vi "Disconnect.vi"(8 "error in":errorcluster, 11 "Luminos in":refnum<class "Luminos.lvclass">) -> (0 "error out":errorcluster, 3 "Luminos out":refnum<class "Luminos.lvclass">)   [LabVIEW 2018, in "Luminos.lvlib" / "Luminos.lvclass"]
uses:
  Luminos.lvclass
  PPLs/Axis/Axis.lvlibp/Axis.lvclass
  <instrlib>/ZaberTSeries/ZaberTSeries.lvlib
  C:/Projects/LabVIEW/PPLs/Axis/Axis.lvlibp/Axis.lvclass
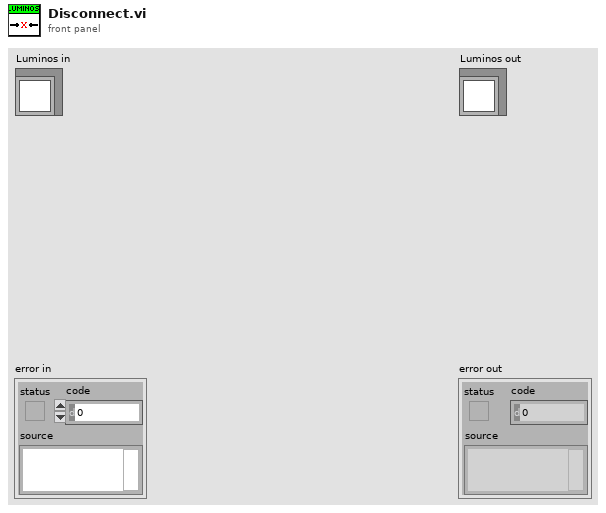
[diagram p1: front panel]
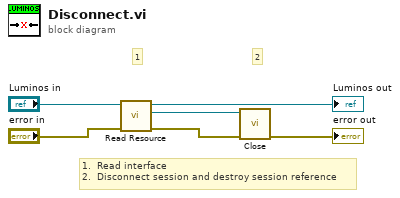
[diagram p0: block diagram]
diagram:
  # "1.  Read interface \n2.  Disconnect session and destroy session reference"
  # "2"
  # "1"
  n1 = call "Read Resource.vi"("error in"="error in", "Axis in"="Luminos in") -> ("error out"=w1:errorcluster, "Resource"=w4:refnum<visa-resource-name>, "Axis out"=→"Luminos out":refnum<class "Luminos.lvclass">)  [unwired: 7 in]
  n2 = call <instrlib>:"Close.vi"("error in (no error)"=w1, "VISA resource name"=w4) -> ("error out"=→"error out":errorcluster)  [unwired: 8 in, 1 out]
